vi "Calculate Target Pose V2.vi"(8 "Robot Calibration Cluster":T2={"Camera Height on robot (in)"=9.5, "Camera Angle on the robot (deg)"=2.5, "Camera FOV Vert View Angle (deg)"=53.5, "Camera FOV Hor View Angle (deg)"=92.0, "Camera Focal Length (mm)"=10.0, "Target size (in)"=6.5, "Distance Correction Factor"=3.952} {"Distance Correction Factor" format="%#_13g"; "Camera FOV Hor View Angle (deg)" format="%#_13g"; "Camera Focal Length (mm)" format="%#_13g"; "Target size (in)" format="%#_13g"; "Camera FOV Vert View Angle (deg)" format="%#_13g"; "Camera Angle on the robot (deg)" format="%#_13g"; "Camera Height on robot (in)" format="%#_13g"}, 9 "Camera Resolution":T3={"Camera Resolution W (pixels)"=800.0, "Camera Resolution H (pixels)"=600.0}, 10 "Corners":cluster{"X":dbl, "Y":dbl}[](array[cluster])=[{"X"=307.872, "Y"=232.024}, {"X"=377.422, "Y"=233.8}, {"X"=378.631, "Y"=168.921}, {"X"=311.507, "Y"=167.884}], 11 "Target Center":cluster{"X":dbl, "Y":dbl}={"X"=343.697, "Y"=200.075}) -> (0 "Homography H":T1, 1 "Roll":dbl, 2 "Pitch":dbl, 3 "Yaw":dbl)   [LabVIEW 2025]
uses:
  Camera Info.ctl
  <vilib>/Analysis/Matrix/Datatypes/RealMatrix.ctl
  <vilib>/Analysis/Matrix/NI_Matrix.lvlib
panel:
  out "VI Execution Time":dbl
  out "World corner points (out)":dbl[][](array[numeric])=[[-3.25, -3.25, 0.0], [3.25, -3.25, 0.0], [3.25, 3.25, 0.0], [-3.25, 3.25, 0.0]]
  out "t Translation Vector":dbl[](array[numeric])
  out "R Rotation Matrix":T1 format="%#_6f"
  out "B Matrix":dbl[][](array[numeric]) format="%#_6f"
  out "Camera intrinsic matrix (K)":dbl[][](array[numeric])=[[-3.25, -3.25, 0.0], [3.25, -3.25, 0.0], [3.25, 3.25, 0.0], [-3.25, 3.25, 0.0]]
  out "half_fov_rad":dbl format="%.5f"
  out "f_px":dbl format="%.5f"
  out "cy height":dbl format="%.5f"
  out "cx width":dbl format="%.5f"
  out "sensor_width_mm/2":dbl format="%.6f"
  out "f_mm":dbl format="%.5f"
  in  "Sensor pixel size (µm)":dbl=3.0
  # "These aare Inputs"
  # "These are calculated values"
  # "Bottom Left"
  # "Bottom Left"
  # "Bottom Right"
  # "Bottom Right"
  # "Top Right"
  # "Top Right"
  # "Top Left"
  # "Top Left"
  # "Bottom Left"
  # "Bottom Right"
  # "Top Right"
  # "Top Left"
  # "Target Center"
  # "Bottom Left"
  # "Bottom Right"
  # "Top Right"
  # "Top Left"
  # "Target Center"
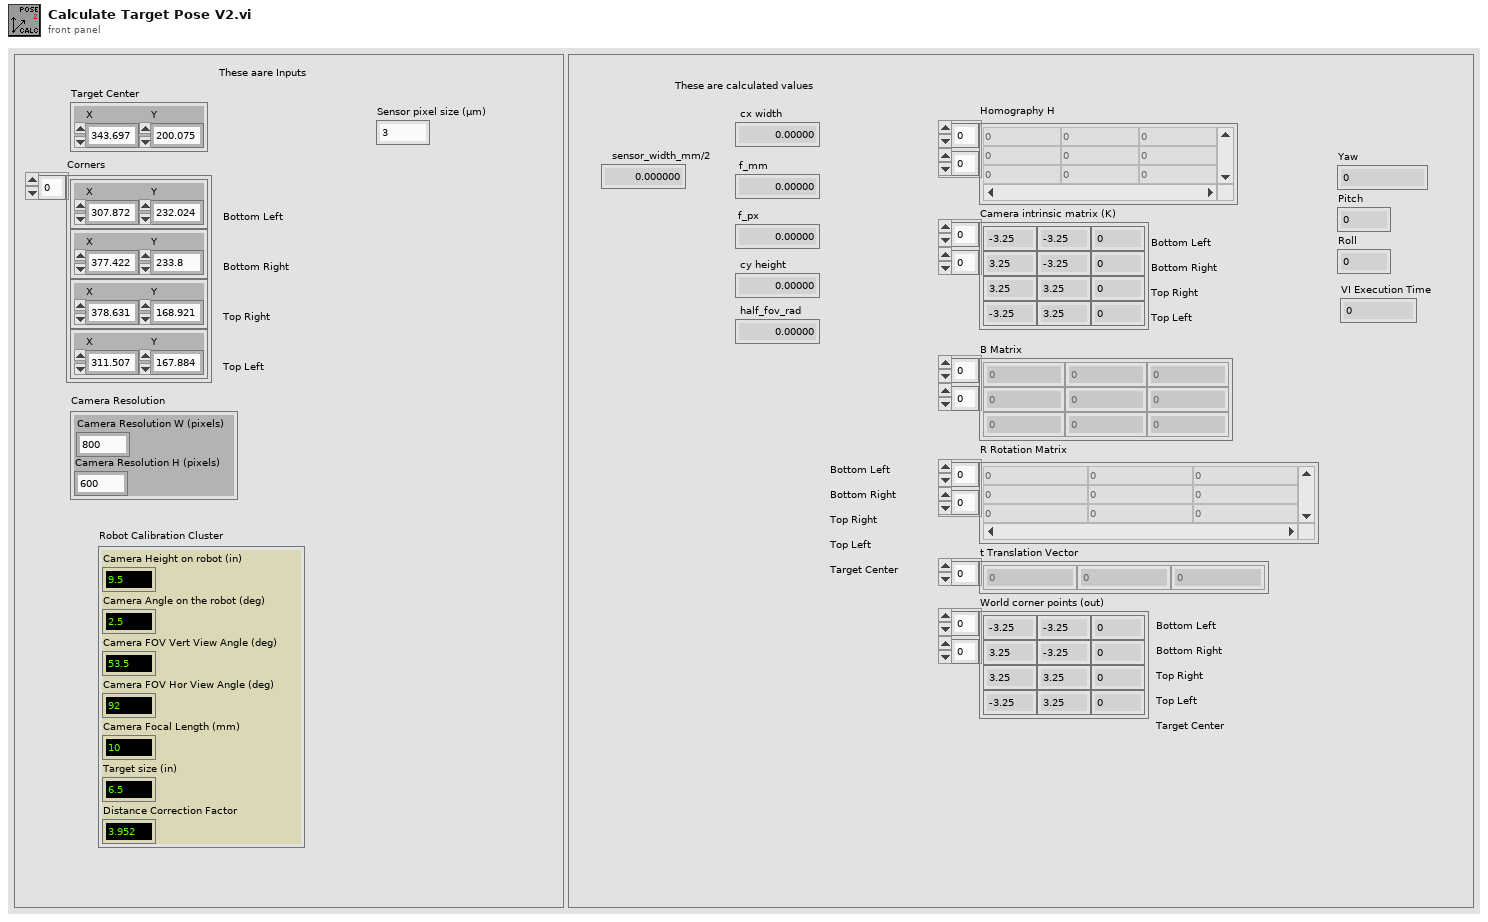
[diagram p1: front panel]
types:
  T1 = typedef "NI_Matrix.lvlib/RealMatrix.ctl" = dbl[][]
  T2 = typedef "Camera Info.ctl" = cluster{"Camera Height on robot (in)":dbl, "Camera Angle on the robot (deg)":dbl, "Camera FOV Vert View Angle (deg)":dbl, "Camera FOV Hor View Angle (deg)":dbl, "Camera Focal Length (mm)":dbl, "Target size (in)":dbl, "Distance Correction Factor":dbl}
  T3 = cluster{"Camera Resolution W (pixels)":dbl, "Camera Resolution H (pixels)":dbl}
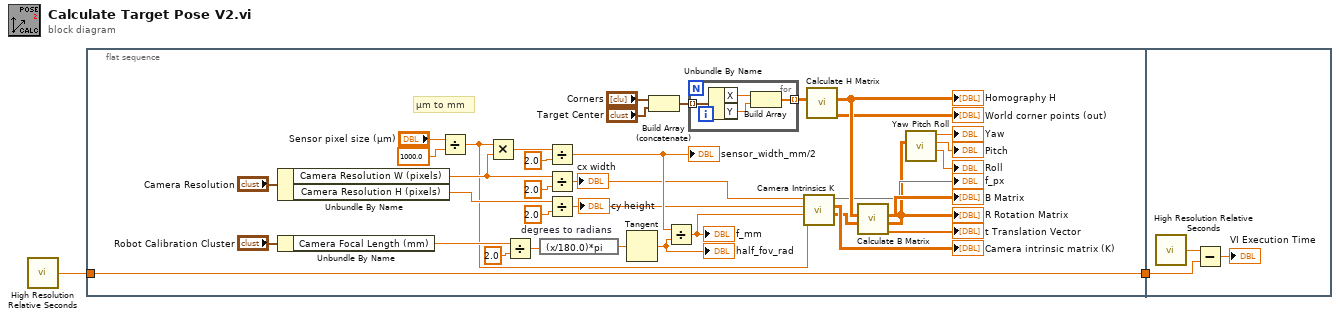
[diagram p0: block diagram]
diagram:
  n1 = call <vilib>:"High Resolution Relative Seconds.vi"() -> ("relative seconds"=w2:dbl)
  n2 = flat-sequence {
    tunnel: w2 -> [w7]
    tunnel: [w7] -> w1
    tunnel: w1 -> [w44]
    frame #0 {
      # "µm to mm"
      n3 = Unbundle By Name("Camera Resolution") -> ("Camera Resolution W (pixels)"=w27:dbl, "Camera Resolution H (pixels)"=w26:dbl)
      n4 = Unbundle By Name("Robot Calibration Cluster") -> ("Camera Focal Length (mm)"=w25:dbl)
      n5 = Divide(x="Sensor pixel size (µm)", y=1000.0) -> (x/y=w18:dbl)
      n6 = Multiply(x=w18, y=w27) -> (x*y=w34:dbl)
      n7 = Divide(x=w25, y=2.0) -> (x/y=w23:dbl)
      n8 = expression code="(x/180.0)*pi" "degrees to radians"(w23) -> (w22:dbl)
      n9 = Divide(x=w34, y=2.0) -> (x/y=w20:dbl)
      "sensor_width_mm/2" <- w20
      n10 = Divide(x=w27, y=2.0) -> (x/y=w9:dbl)
      "cx width" <- w9
      n11 = Divide(x=w26, y=2.0) -> (x/y=w8:dbl)
      "cy height" <- w8
      n12 = Tangent(1:w22) -> (0:w21:dbl)
      "half_fov_rad" <- w21
      n13 = Build Array (concatenate)("Corners", "Target Center") -> (w29:cluster{"X":dbl, "Y":dbl}[])
      n14 = Divide(x=w20, y=w21) -> (x/y=w19:dbl)
      "f_mm" <- w19
      n15 = for {
        tunnel: w29 -> [w42] mode=indexing
        tunnel: [w39] -> w13 mode=indexing
        n16 = Unbundle By Name(w42) -> ("X"=w41:dbl, "Y"=w40:dbl)
        n17 = Build Array(w41, w40) -> (w39:dbl[])
      }
      n18 = call "Camera Intrinsics K.vi"(8:w18, "Robot Calibration Cluster"=w19, "Picture Cluster"=w8, 11:w9) -> ("Camera intrinsic matrix (K^-1)"=w15:dbl[][], "Camera intrinsic matrix (K)"=→"Camera intrinsic matrix (K)":dbl[][], 3:→"f_px")  [unwired: 5 in]
      n19 = call "Calculate H Matrix.vi"("Measured Points"=w13) -> ("World corner points (out)"=→"World corner points (out)":dbl[][], "Homography H"=w16:T1)  [unwired: 8 in, 1 out]
      "Homography H" <- w16
      n20 = call "Calculate B Matrix.vi"("Camera intrinsic matrix (K^-1)"=w15, "Homography H"=w16) -> ("t (Translation Vector)"=→"t Translation Vector":dbl[], "R Rotation Matrix (final)"=w6:T1, "B Matrix"=→"B Matrix":dbl[][])  [unwired: 7 in]
      "R Rotation Matrix" <- w6
      n21 = call "Yaw Pitch Roll.vi"("R Rotation Matrix"=w6) -> ("Roll"=→"Roll":dbl, "Pitch"=→"Pitch":dbl, "Yaw"=→"Yaw":dbl)  [unwired: 8 in]
    }
    frame #1 {
      n22 = call <vilib>:"High Resolution Relative Seconds.vi"() -> ("relative seconds"=w45:dbl)
      n23 = Subtract(x=w45, y=w44) -> (x-y=→"VI Execution Time":dbl)
    }
  }
